vi "JoystickSquared.vi"(10 "Joystick Value":dbl) -> (2 "Joystick Value Squared":dbl)   [LabVIEW 2014]
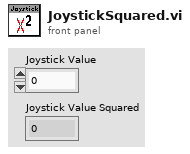
[diagram p1: front panel]
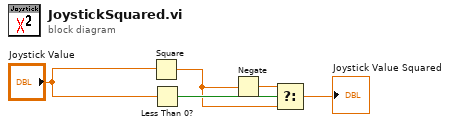
[diagram p0: block diagram]
diagram:
  n1 = Square(x="Joystick Value") -> (x^2=w4:dbl)
  n2 = Less Than 0?(x="Joystick Value") -> (x < 0?=w5:bool)
  n3 = Negate(x=w4) -> (-x=w3:dbl)
  n4 = Select(t=w3, s=w5, f=w4) -> (s? t:f=→"Joystick Value Squared":dbl)
